vi "Dynamic_dispatch.vi"() -> ()   [LabVIEW 2017]
doc: "Demonstrates dynamic dispatching with LabVIEW classes."
uses:
  Square/Square.lvclass
  C:/Users/smallesh/Documents/FINALE.typescript/src/testAssets/disabled/Dynamic_dispatch/Shape/Shape.lvclass
  Shape/Shape.lvclass
  Triangle/Triangle.lvclass
panel:
  out "names":string[](array[string])
  # "Overview: Demonstrates dynamic dispatching with LabVIEW classes.\nInstructions:\n1. Run the VI to see the list of LabVIEW class names.\n2. Open the block diagram and refer to the comments there."
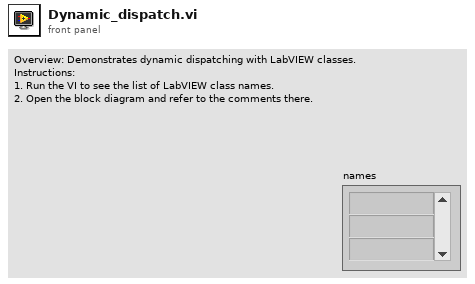
[diagram p1: front panel]
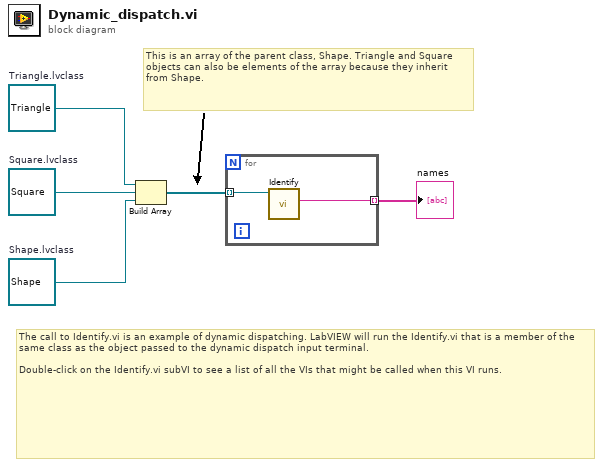
[diagram p0: block diagram]
diagram:
  w1 = refnum<class "Triangle.lvclass"> refnum  # Triangle.lvclass
  w2 = refnum<class "Shape.lvclass"> refnum  # Shape.lvclass
  w3 = refnum<class "Square.lvclass"> refnum  # Square.lvclass
  # "This is an array of the parent class, Shape. Triangle and Square objects can also be elements of the array because they inherit from Shape."
  # "The call to Identify.vi is an example of dynamic dispatching. LabVIEW will run the Identify.vi that is a member of the same class as the object passed to the dynamic dispatch input terminal.\n\nDouble-click on the Identify.vi subVI to see a list of all the VIs that might be called when this VI runs."
  n1 = Build Array(w1, w3, w2) -> (w5:refnum<class "Shape.lvclass">[])
  n2 = for {
    tunnel: w5 -> [w7] mode=indexing
    tunnel: [w6] -> w4 mode=indexing
    n3 = call-dynamic "Identify.vi"("Shape in"=w7) -> ("Class name"=w6:string)  [unwired: 8 in, 2 out]
  }
  "names" <- w4
